vi "Processing Step.vi"(8 "error in (no error)":errorcluster, 11 "Exception Handler in":refnum<class "Exception Handler.lvclass">) -> (0 "error out":errorcluster, 2 "Step":T1[](array[typedef]), 3 "Exception Handler out":refnum<class "Exception Handler.lvclass">)   [LabVIEW 2020, in "HTTP Server.lvlib" / "Exception Handler.lvclass"]
uses:
  Exception Handler.lvclass
  Processing Step.ctl
  HTTP Server.lvlib
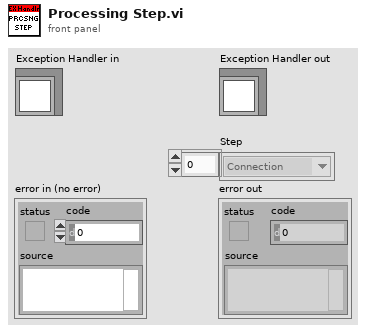
[diagram p1: front panel]
types:
  T1 = typedef "HTTP Server.lvlib/Processing Step.ctl" = enum16{"Connection", "Request", "Routing", "Controller Init", "Controller", "Response", "Cleanup", "Exception"}
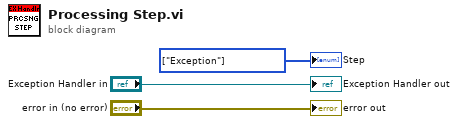
[diagram p0: block diagram]
diagram:
  w1 = T1[] [enum."Exception"] items=["Connection", "Request", "Routing", "Controller Init", "Controller", "Response", "Cleanup", "Exception"] ("Array")
  "error out" <- "error in (no error)"
  "Exception Handler out" <- "Exception Handler in"
  "Step" <- w1
